vi "Read Heater Output Data.vi"(8 "error in (no error)":errorcluster, 11 "VISA resource name":refnum<visa-resource-name>) -> (0 "error out":errorcluster, 2 "Heater Output":dbl min=0.0 max=100.0 step=1e-05 format="%^.5e", 3 "VISA resource name out":refnum<visa-resource-name>)   [LabVIEW 2015, in "Lake Shore 372.lvlib"]
doc: "Returns the heater output in percent of current or in actual power depending on the heater output selection. This VI uses the <B>HTR?</B> command.\n\nNote: This only applies to the sample heater, use <B>AOUT?</B> for the warm-up heater and the analog/still output."
uses:
  <instrlib>/Lake Shore 372/Lake Shore 372.lvlib
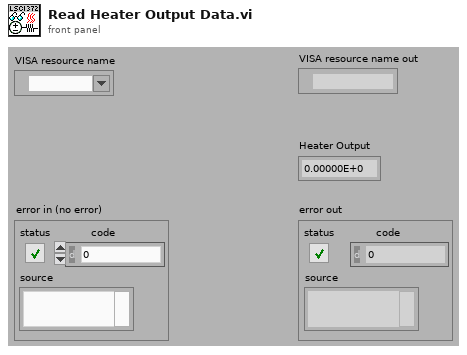
[diagram p1: front panel]
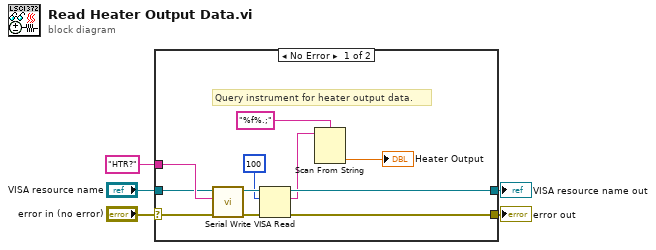
[diagram p0: block diagram]
diagram:
  n1 = case shown="No Error" "error in (no error)" {
    selector: "error in (no error)" -> [w7 w17]
    tunnel: "HTR?" -> [w13 _]
    tunnel: "VISA resource name" -> [w12 w18]
    tunnel: [w11 w17] -> w3
    tunnel: [w10 w18] -> w2
    frame No Error {
      # "Query instrument for heater output data."
      n2 = call <instrlib>:"Serial Write.vi"("error in (no error)"=w7, "Write Buffer (\"\")"=w13, "VISA resource name"=w12) -> ("error out"=w15:errorcluster, "VISA resource name out"=w16:refnum<visa-resource-name>)  [unwired: 6 in, 1 out]
      n3 = VISA Read(VISA resource name=w16, byte count=100, error in (no error)=w15) -> (VISA resource name out=w10:refnum<visa-resource-name>, read buffer=w6:string, error out=w11:errorcluster)  [unwired: 1 out]
      n4 = Scan From String(format string="%f%.;", input string=w6) -> (output 1=→"Heater Output":dbl)  [unwired: 3 in, 3 out]
    }
    frame Error {
    }
  }
  "error out" <- w3
  "VISA resource name out" <- w2
